vi "Initalise spectrometer.vi"(10 "Continous strobe delay":i32, 11 "Enter the \nInetegration Time":i32) -> (0 "Wrapper Out":u32, 2 "ContinuousStrobe Out":u32, 3 "WL Values":dbl[](array[numeric]))   [LabVIEW 2020]
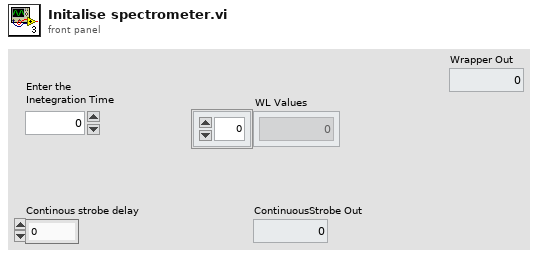
[diagram p1: front panel]
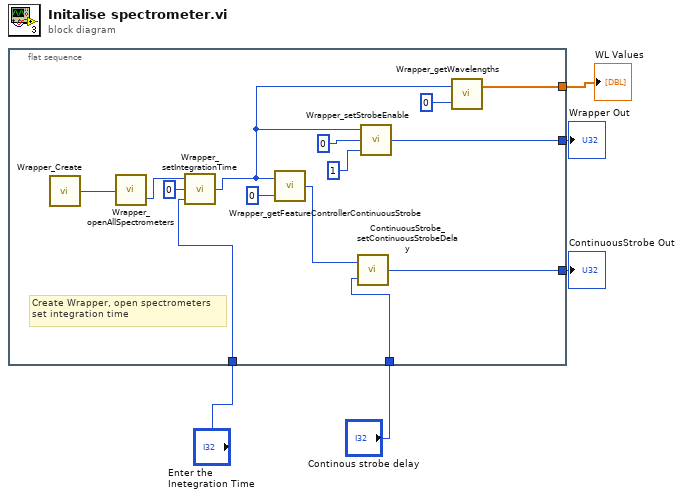
[diagram p0: block diagram]
diagram:
  n1 = flat-sequence {
    tunnel: "Enter the \nInetegration Time" -> [w9]
    tunnel: [w10] -> w5
    tunnel: "Continous strobe delay" -> [w8]
    tunnel: [w7] -> w4
    tunnel: [w6] -> w1
    frame #0 {
      # "Create Wrapper, open spectrometers\nset integration time"
      n2 = call "Wrapper_Create.vi"() -> ("Wrapper"=w19:u32)
      n3 = call "Wrapper_openAllSpectrometers.vi"("Wrapper In"=w19) -> ("Wrapper Out"=w13:u32)  [unwired: 1 out]
      n4 = call "Wrapper_setIntegrationTime.vi"("Integration Time"=w9, "Spectrometer Index"=0 ("Index"), "Wrapper In"=w13) -> ("Wrapper Out"=w11:u32)
      n5 = call "Wrapper_getFeatureControllerContinuousStrobe.vi"("Index"=0, "Wrapper"=w11) -> ("ContinuousStrobe"=w16:u32)
      n6 = call "ContinuousStrobe_setContinuousStrobeDelay.vi"("delay"=w8, "ContinuousStrobe In"=w16) -> ("ContinuousStrobe Out"=w7:u32)
      n7 = call "Wrapper_setStrobeEnable.vi"("On/Off"=1, "Index"=0, "Wrapper In"=w11) -> ("Wrapper Out"=w6:u32)
      n8 = call "Wrapper_getWavelengths.vi"("Index"=0, "Wrapper"=w11) -> ("WL Values"=w10:dbl[])  [unwired: 1 out]
    }
  }
  "ContinuousStrobe Out" <- w4
  "WL Values" <- w5
  "Wrapper Out" <- w1
